vi "incerc_si_incerc.vi"() -> ()   [LabVIEW 2015]
uses:
  <vilib>/imath/engines/lvmath2/RunTimeEngine/RangeToken/NIMS_Range_R2 - Integer.vi
  <instcachedir>/0/NIMS_Range_R2 - Integer_396D5D4FB869421F9245109A0975AD54.lvgen/NIMS_Range_R2 - Integer_396D5D4FB869421F9245109A0975AD54_000.vi
  <vilib>/imath/engines/lvmath2/RunTimeEngine/CommandStatement/MC_CommandStatement_break.vi
  <vilib>/imath/engines/lvmath2/RunTimeEngine/IndexRead/NIMS M(S,S).vi
  <instcachedir>/0/NIMS M(S,S)_AC51E74150A542F7991B9634C66F3096.lvgen/NIMS M(S,S)_AC51E74150A542F7991B9634C66F3096_003.vi
  <vilib>/imathl/engines/lvmath/Functions/Error Handling/Create Error.vi
  <vilib>/imath/engines/lvmath2/RunTimeEngine/IndexReplace/NIMS M(S,S)=S.vi
  <instcachedir>/0/NIMS M(S,S)=S_72298AC072A24B679F5E0C14DB2DD503.lvgen/NIMS M(S,S)=S_72298AC072A24B679F5E0C14DB2DD503_002.vi
  <vilib>/imath/engines/lvmath2/RunTimeEngine/ErrorHandling/NIMS_Finalize Error.vi
panel:
  out "initialized array":i8[][](array[numeric])
  in  "Path":path
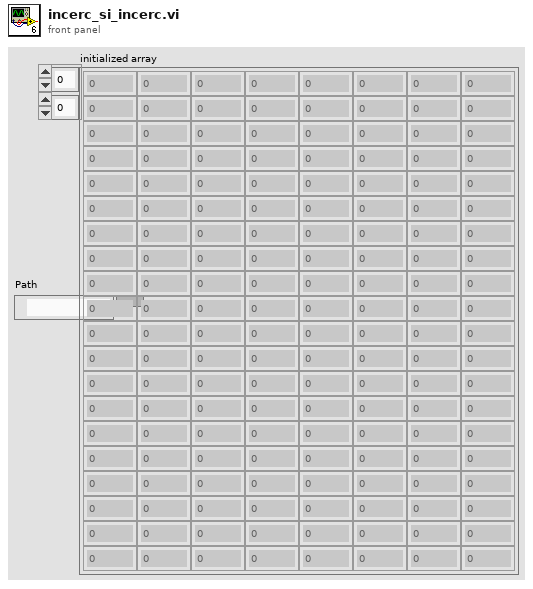
[diagram p1: front panel]
types:
  T1 = typedef "imagedata.ctl" = cluster{"image type":i32, "image depth":i32, "image":u8[], "mask":u8[], "colors":u32[], "Rectangle":cluster{"left":i16, "top":i16, "right":i16, "bottom":i16}}
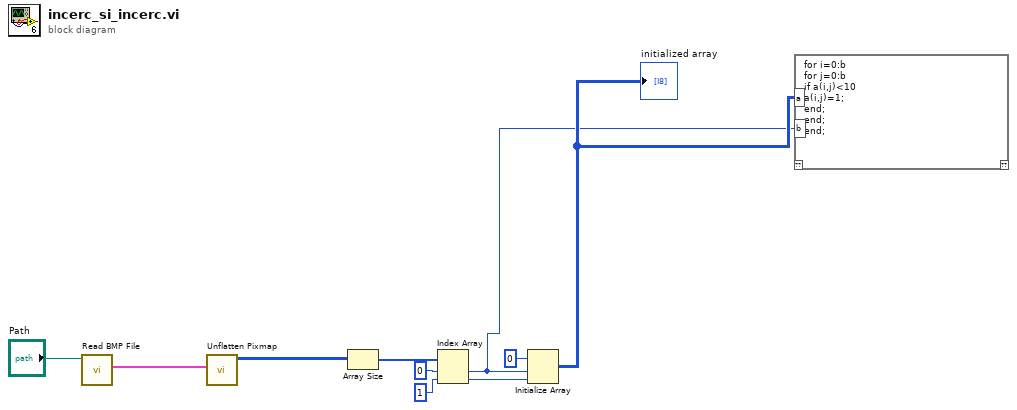
[diagram p0: block diagram]
diagram:
  n1 = call <vilib>:"Read BMP File.vi"("path to BMP file"="Path") -> ("image data"=w9:T1)  [unwired: 8 in, 2 out]
  n2 = call <vilib>:"Unflatten Pixmap.vi"("image data"=w9) -> ("24-bit pixmap"=w3:u32[][])  [unwired: 4 in, 6 out]
  n3 = Array Size(array=w3) -> (size(s)=w8:i32[])
  n4 = Index Array(array=w8, index #1=0 ("index"), index #2=1 ("index")) -> (element #1=w1:i32, element #2=w5:i32)
  n5 = Initialize Array(i8 0 ("element"), w1, w5) -> (w2:i8[][])
  "initialized array" <- w2
  n6 = mathscript code="for i=0:b\nfor j=0:b\nif a(i,j)<10\na(i,j)=1;\nend;\nend;\nend;"("a"=w2, "b"=w1) -> ()  [unwired: 1 in, 1 out]
